vi "SeqRead.vi"(8 "error in (no error)":errorcluster, 11 "File in Refnum":refnum<file>) -> (0 "error out":errorcluster, 1 "Cohort List":cluster{string, i32}[](array[cluster]), 2 "SEQ out":refnum<class "Sequence.lvclass">, 3 "File out Refnum":refnum<file>)   [LabVIEW 2012, in "Sequence.lvclass"]
uses:
  Sequence.lvclass
  Cohort.lvclass
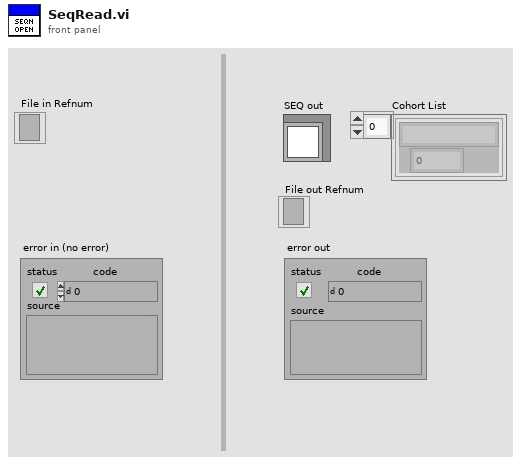
[diagram p1: front panel]
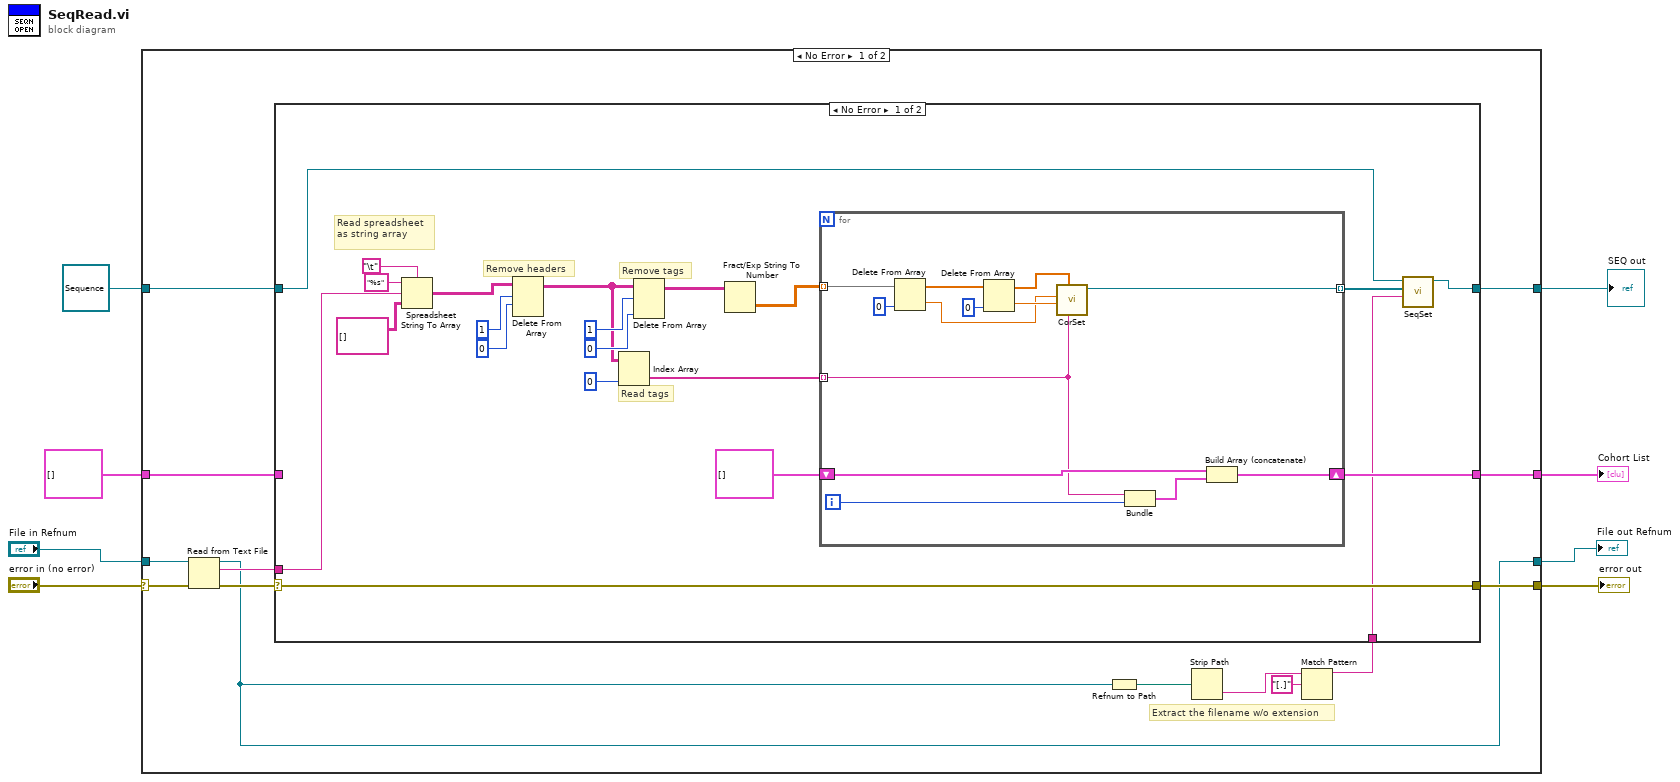
[diagram p0: block diagram]
diagram:
  n1 = case shown="No Error" "error in (no error)" {
    selector: "error in (no error)" -> [w19 w63]
    tunnel: [w20 w63] -> w7
    tunnel: [w18 w61] -> w6
    tunnel: [w17 w62] -> w5
    tunnel: cluster{string, i32}[] [] -> [w16 w62]
    tunnel: refnum<class "Sequence.lvclass"> refnum ("Sequence.lvclass") -> [w15 w61]
    tunnel: [w13 w60] -> w2
    tunnel: "File in Refnum" -> [w9 w60]
    frame No Error {
      # "Extract the filename w/o extension"
      n2 = Read from Text File(file (use dialog)=w9, error in=w19) -> (refnum out=w13:refnum<file>, text=w22:string, error out=w21:errorcluster)  [unwired: 2 in, 1 out]
      n3 = Refnum to Path(1:w13) -> (0:w14:path)
      n4 = Strip Path(path=w14) -> (name=w12:string)  [unwired: 1 out]
      n5 = Match Pattern(string=w12, regular expression="[.]") -> (before substring=w10:string)  [unwired: 1 in, 3 out]
      n6 = case shown="No Error" w21 {
        selector: w21 -> [w40 w59]
        tunnel: [w43 w58] -> w17
        tunnel: w22 -> [w41 _]
        tunnel: [w34 w57] -> w18
        tunnel: [w40 w59] -> w20
        tunnel: w16 -> [_ w58]
        tunnel: w15 -> [w23 w57]
        tunnel: w10 -> [w24 _]
        frame No Error {
          # "Remove tags"
          # "Read tags"
          # "Remove headers"
          # "Read spreadsheet as string array"
          n7 = Spreadsheet String To Array(delimiter (Tab)="\t", format string="%s", spreadsheet string=w41, array type (2D Dbl)=string[][] []) -> (array=w37:string[][])
          n8 = Delete From Array(array=w37, length=1, index (row)=0) -> (array with subset deleted=w27:string[][])  [unwired: 1 in, 1 out]
          n9 = Index Array(array=w27, index (col)=0 ("disabled index (col)")) -> (element=w26:string[])  [unwired: 1 in]
          n10 = Delete From Array(array=w27, length=1, index (col)=0 ("index (row)")) -> (array with subset deleted=w32:string[][])  [unwired: 1 in, 1 out]
          n11 = Fract/Exp String To Number(string=w32) -> (number=w36:dbl[][])  [unwired: 3 in, 1 out]
          n12 = for {
            shift-right: [w56] -> w43
            shift-left: cluster{string, i32}[] [] -> [w55]
            tunnel: w36 -> [w52] mode=indexing
            tunnel: [w48] -> w35 mode=indexing
            tunnel: w26 -> [w44] mode=indexing
            i -> [w53]
            n13 = Delete From Array(array=w52, index=0) -> (deleted portion=w45:dbl, array with subset deleted=w49:dbl[])  [unwired: 1 in]
            n14 = Delete From Array(array=w49, index=0) -> (deleted portion=w47:dbl, array with subset deleted=w46:dbl[])  [unwired: 1 in]
            n15 = call "CorSet.vi"("Set COR Tag"=w44, "Set Electrodes"=w46, "Set Pulse Width"=w47, "Set Pulse Frequency"=w45) -> ("Cohort out"=w48:refnum<class "Cohort.lvclass">)  [unwired: 6 in, 1 out]
            n16 = Bundle(w44, w53) -> (w54:cluster{string, i32})  [unwired: 1 in]
            n17 = Build Array (concatenate)(w55, w54) -> (w56:cluster{string, i32}[])
          }
          n18 = call "SeqSet.vi"("Tag"=w24, "Array of COR"=w35, "SEQ in"=w23) -> ("SEQ out"=w34:refnum<class "Sequence.lvclass">)  [unwired: 7 in, 1 out]
        }
        frame Error {
        }
      }
    }
    frame Error {
    }
  }
  "error out" <- w7
  "SEQ out" <- w6
  "Cohort List" <- w5
  "File out Refnum" <- w2
